vi "Set to HOME.vi"(0 "Zaber":T1={"Serial port handle"="", "Axis"="", "Controller #"=0, "Min position"=0.0, "Max position"=0.0, "Min velocity"=0.0, "Max velocity"=0.0, "Firmware"="", "Device ID"=0, "Variable event"=refnum, "Variable ref"=refnum, "Resolution, usteps/step"=0, "Serial port semaphore"=refnum, "Joystick buttons"={"MinDir"=1, "MaxDir"=2, "MedSpeed"=5, "HighSpeed"=6}} {"Joystick buttons"."HighSpeed" min=1 max=25 step=1; "Joystick buttons"."MedSpeed" min=1 max=25 step=1; "Joystick buttons"."MaxDir" min=1 max=25 step=1; "Joystick buttons"."MinDir" min=1 max=25 step=1}, 5 "error in":errorcluster) -> (14 "Zaber out":T1={"Serial port handle"="", "Axis"="", "Controller #"=0, "Min position"=0.0, "Max position"=0.0, "Min velocity"=0.0, "Max velocity"=0.0, "Firmware"="", "Device ID"=0, "Variable event"=refnum, "Variable ref"=refnum, "Resolution, usteps/step"=0, "Serial port semaphore"=refnum, "Joystick buttons"={"MinDir"=1, "MaxDir"=2, "MedSpeed"=5, "HighSpeed"=6}} {"Joystick buttons"."HighSpeed" min=1 max=25 step=1; "Joystick buttons"."MedSpeed" min=1 max=25 step=1; "Joystick buttons"."MaxDir" min=1 max=25 step=1; "Joystick buttons"."MinDir" min=1 max=25 step=1}, 19 "error out":errorcluster)   [LabVIEW 2018]
uses:
  Zaber.ctl
  GenericDataEvent/GenericEvent.ctl
  ZaberVariables.ctl
  CommandZaber.ctl
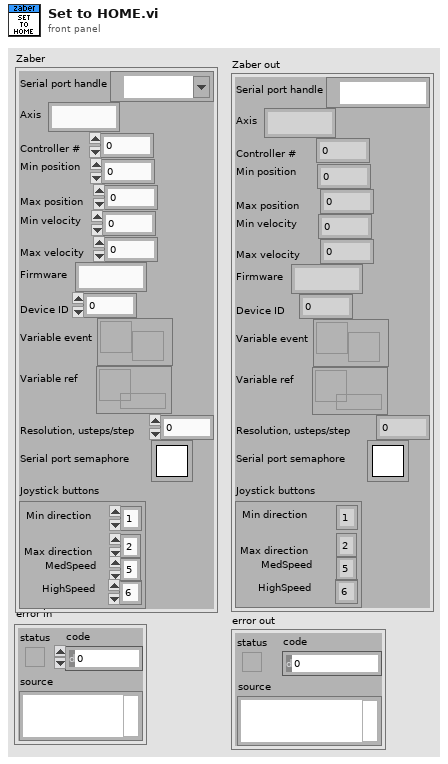
[diagram p1: front panel]
types:
  T1 = typedef "Zaber.ctl" = cluster{"Serial port handle":refnum<visa-resource-name>, "Axis":string, "Controller #":u8, "Min position":dbl, "Max position":dbl, "Min velocity":dbl, "Max velocity":dbl, "Firmware":string, "Device ID":i32, "Variable event":T2, "Variable ref":refnum<data-value>, "Resolution, usteps/step":i32, "Serial port semaphore":T3, "Joystick buttons":cluster{"MinDir":i32, "MaxDir":i32, "MedSpeed":i32, "HighSpeed":i32}}
  T2 = typedef "GenericEvent.ctl" = refnum<user-event>
  T3 = typedef "Semaphore RefNum" = refnum<k1>
  T4 = typedef "CommandZaber.ctl" = cluster{"Command":u8, "Data":i32}
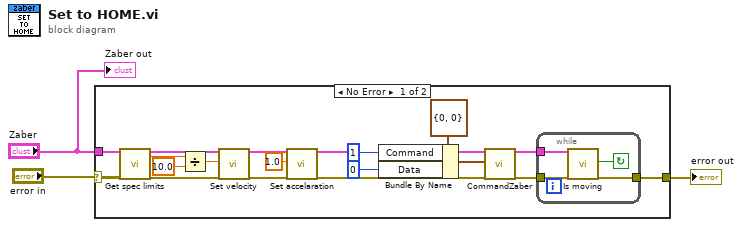
[diagram p0: block diagram]
diagram:
  n1 = case shown="No Error" "error in" {
    selector: "error in" -> [w13 w27]
    tunnel: [w16 w27] -> w2
    tunnel: "Zaber" -> [w12 _]
    frame No Error {
      n2 = call "Get spec limits.vi"("Zaber"=w12, "error in"=w13) -> ("Zaber out"=w10:T1, "MAX velocity, mm/s"=w8:dbl, "error out"=w11:errorcluster)  [unwired: 13 in, 2 out]
      n3 = Divide(x=w8, y=10.0) -> (x/y=w9:dbl)
      n4 = call "Set velocity.vi"("Zaber in"=w10, "Velocity, mm/s"=w9, "error in"=w11) -> ("Zaber out"=w4:T1, "error out"=w5:errorcluster)  [unwired: 14 in, 1 out]
      n5 = call "Set accelaration.vi"("Zaber in"=w4, "Acceration, mm/s/s"=1.0, "error in"=w5) -> ("Zaber out"=w18:T1, "error out"=w17:errorcluster)  [unwired: 13 in, 2 out]
      n6 = Bundle By Name(cluster=T4 {"Command"=0, "Data"=0} ("Command"), "Command"=1 ("Data"), "Data"=0) -> (w21:T4)
      n7 = call "CommandZaber.vi"("Zaber"=w18, "Command"=w21, "error in"=w17) -> ("Zaber out"=w15:T1, "error out"=w14:errorcluster)  [unwired: 13 in, 2 out]
      n8 = while {
        tunnel: w14 -> [w26]
        tunnel: [w24] -> w16
        tunnel: w15 -> [w25]
        stop <- w23 continue-if-true
        n9 = call "Is moving.vi"("Zaber"=w25, "error in"=w26) -> ("Is moving?"=w23:bool, "error out"=w24:errorcluster)  [unwired: 14 in, 2 out]
      }
    }
    frame Error {
    }
  }
  "error out" <- w2
  "Zaber out" <- "Zaber"
